vi "mqttCmdConnectClassWrite.vi"(0 "mqttConnect in":refnum<class "mqttCmdConnect.lvclass">, 5 "mqtt.lvclass":refnum<class "mqtt.lvclass">, 11 "error in (no error)":errorcluster) -> (4 "mqttConnect out":refnum<class "mqttCmdConnect.lvclass">, 15 "error out":errorcluster)   [LabVIEW 2013, in "mqttCmdConnect.lvclass"]
uses:
  mqttCmdConnect.lvclass
  mqtt.lvclass
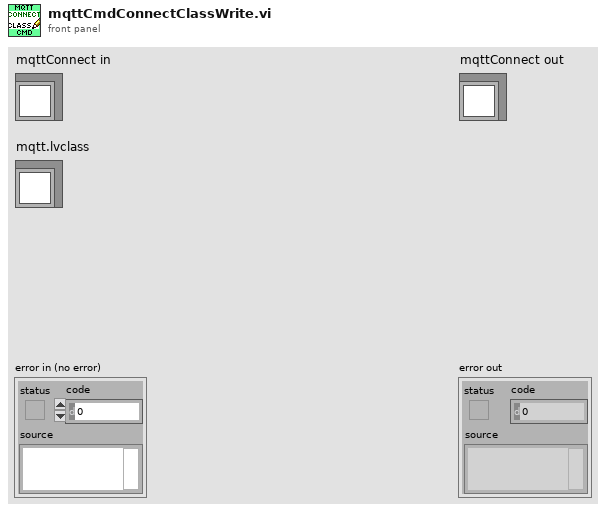
[diagram p1: front panel]
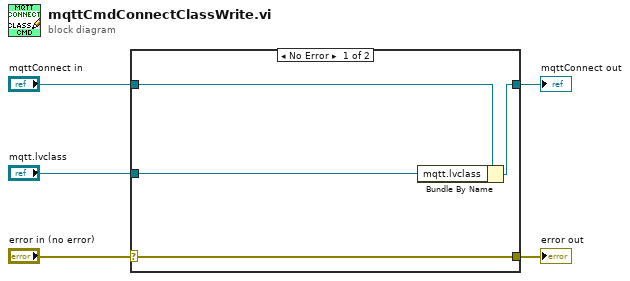
[diagram p0: block diagram]
diagram:
  n1 = case shown="No Error" "error in (no error)" {
    selector: "error in (no error)" -> [w9 w10]
    tunnel: [w9 w10] -> w4
    tunnel: [w7 w11] -> w2
    tunnel: "mqttConnect in" -> [w8 w11]
    tunnel: "mqtt.lvclass" -> [w6 _]
    frame No Error {
      n2 = Bundle By Name(cluster=w8, "mqtt.lvclass"=w6) -> (w7:refnum<class "mqttCmdConnect.lvclass">)
    }
    frame Error {
    }
  }
  "error out" <- w4
  "mqttConnect out" <- w2
